vi "Read DoorParams.vi"(8 "error in (no error)":errorcluster, 11 "Door":refnum<class "Door.lvclass">) -> (0 "error out":errorcluster, 2 "DoorParams":T1, 3 "Door":refnum<class "Door.lvclass">)   [LabVIEW 2020, in "Door.lvclass"]
uses:
  Door.lvclass
  TypeDef/DoorParams.ctl
  Room/Room.lvclass
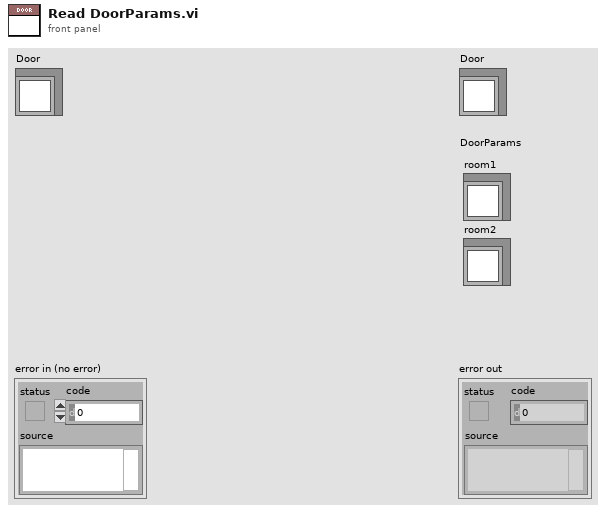
[diagram p1: front panel]
types:
  T1 = typedef "Door.lvclass/DoorParams.ctl" = cluster{"room1":refnum<class "Room.lvclass">, "room2":refnum<class "Room.lvclass">}
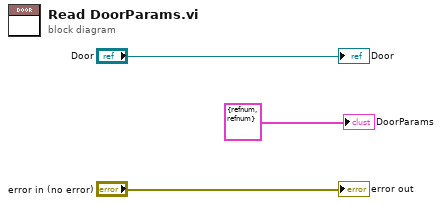
[diagram p0: block diagram]
diagram:
  "error out" <- "error in (no error)"
  "Door" <- "Door"
  "DoorParams" <- T1 {"room1"=refnum, "room2"=refnum} ("<ClassName>Params")
